vi "Acquisition_pluviometrie.vi"() -> ()   [LabVIEW 2017]
panel:
  out "x/y":dbl
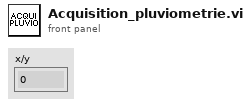
[diagram p1: front panel]
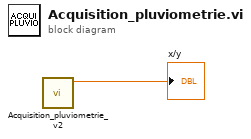
[diagram p0: block diagram]
diagram:
  n1 = call "Acquisition_pluviometrie_v2.vi"() -> ("Numérique"=→"x/y":dbl)  [unwired: 11 in]
